vi "Setup Statically-Linked subWorkers.vi"(8 "error in":errorcluster, 11 "Controller in":refnum<class "Controller.lvclass">) -> (0 "error out":errorcluster, 3 "Controller out":refnum<class "Controller.lvclass">)   [LabVIEW 2024, in "Controller.lvclass"]
doc: "This VI performs a setup of all the statically-linked subWorkers that belong to the Worker that owns this VI. This VI must be called <b>before</b> any statically-linked subWorkers are called."
uses:
  Controller.lvclass
  Controller.lvclass/Controller.ctl
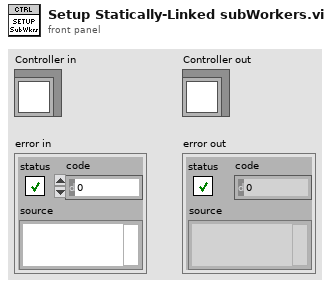
[diagram p1: front panel]
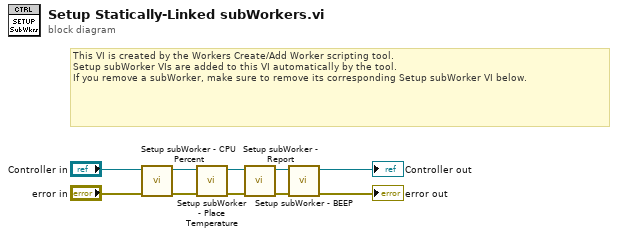
[diagram p0: block diagram]
diagram:
  # "This VI is created by the Workers Create/Add Worker scripting tool.\nSetup subWorker VIs are added to this VI automatically by the tool.\nIf you remove a subWorker, make sure to remove its corresponding Setup subWorker VI below."
  n1 = call "Setup subWorker - CPU Percent.vi"("error in"="error in", "Controller in"="Controller in") -> ("error out"=w9:errorcluster, "Controller out"=w6:refnum<class "Controller.lvclass">)  [unwired: 8 in]
  n2 = call "Setup subWorker - Place Temperature.vi"("error in"=w9, "Controller in"=w6) -> ("error out"=w7:errorcluster, "Controller out"=w4:refnum<class "Controller.lvclass">)  [unwired: 8 in]
  n3 = call "Setup subWorker - Report.vi"("error in"=w7, "Controller in"=w4) -> ("error out"=w5:errorcluster, "Controller out"=w3:refnum<class "Controller.lvclass">)  [unwired: 8 in]
  n4 = call "Setup subWorker - BEEP.vi"("error in"=w5, "Controller in"=w3) -> ("error out"=→"error out":errorcluster, "Controller out"=→"Controller out":refnum<class "Controller.lvclass">)  [unwired: 8 in]
